vi "Configure Timer.vi"(8 "error in (no error)":errorcluster, 10 "Internal timer (2 s)":dbl=2.0, 11 "VISA resource name":refnum<visa-resource-name>) -> (0 "error out":errorcluster, 3 "VISA resource name out":refnum<visa-resource-name>)   [LabVIEW 2020, in "QuPMXdriver.lvlib"]
doc: "Configures internal timer. Input value is in seconds, resolution to miliseconds (given by multiplexer)."
uses:
  QuPMXdriver.lvlib
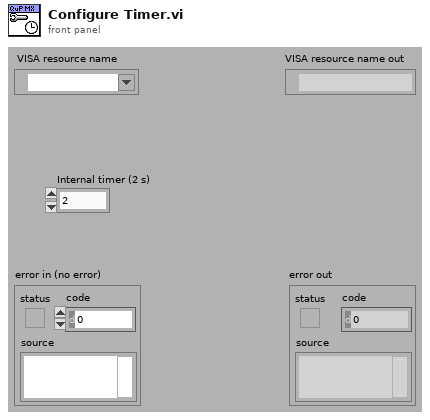
[diagram p1: front panel]
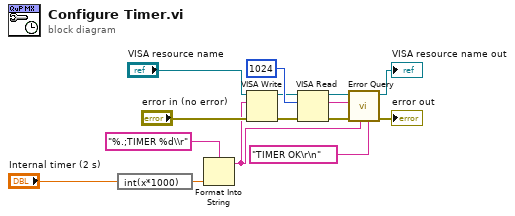
[diagram p0: block diagram]
diagram:
  n1 = expression code="int(x*1000)"("Internal timer (2 s)") -> (w9:dbl)
  n2 = Format Into String(format string="%.;TIMER %d\\r", w9) -> (resulting string=w3:string)  [unwired: 2 in, 1 out]
  n3 = VISA Write(VISA resource name="VISA resource name", write buffer=w3, error in (no error)="error in (no error)") -> (VISA resource name out=w6:refnum<visa-resource-name>, error out=w1:errorcluster)  [unwired: 1 out]
  n4 = VISA Read(VISA resource name=w6, byte count=u32 1024, error in (no error)=w1) -> (VISA resource name out=w7:refnum<visa-resource-name>, read buffer=w5:string, error out=w4:errorcluster)  [unwired: 1 out]
  n5 = call "Error Query.vi"("Expected read buffer"="TIMER OK\r\n" ("read buffer"), "Last command"=w3, "error in (no error)"=w4, "Read buffer"=w5, "VISA resource name"=w7) -> ("error out"=→"error out":errorcluster, "VISA resource name out"=→"VISA resource name out":refnum<visa-resource-name>)  [unwired: 5 in]
